vi "LEIN m serial Open Comport.vi"(0 "Comport":refnum<visa-resource-name>, 9 "baud rate (9600)":u32=9600, 11 "error in (no error)":errorcluster, 13 "Reply timeout (1000 ms)":u32=1000) -> (4 "VISA resource name out":refnum<visa-resource-name>, 15 "error out":errorcluster)   [LabVIEW 2011]
doc: "Opner comporten med den valgte VISA ingangen, om error in, gjøre ingenting"
uses:
  <vilib>/Instr/_visa.llb/VISA Configure Serial Port (Instr).vi
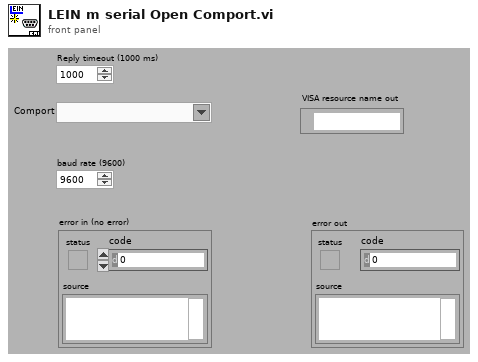
[diagram p1: front panel]
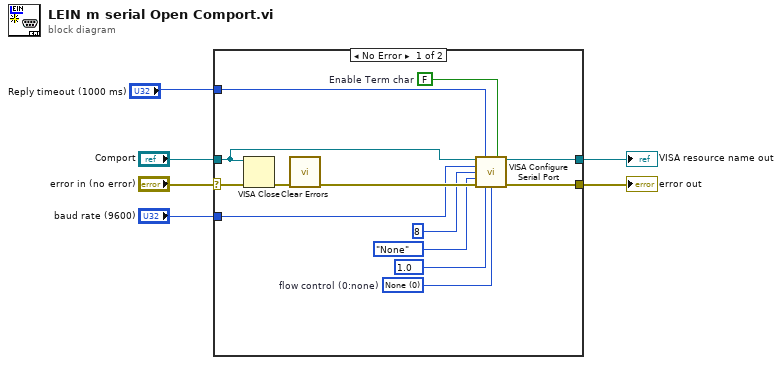
[diagram p0: block diagram]
diagram:
  n1 = case shown="No Error" "error in (no error)" {
    selector: "error in (no error)" -> [w15 w20]
    tunnel: [w18 w21] -> w6
    tunnel: [w17 w20] -> w5
    tunnel: "Comport" -> [w12 w21]
    tunnel: "Reply timeout (1000 ms)" -> [w11 _]
    tunnel: "baud rate (9600)" -> [w10 _]
    frame No Error {
      w9 = u16 10 items=["1.0"=10, "1.5"=15, "2.0"=20] ("stop bits (10: 1 bit)")
      w19 = FALSE  # Enable Term char
      w16 = u16 0 items=["None", "XON/XOFF", "RTS/CTS", "XON/XOFF & RTS/CTS", "DTR/DSR", "XON/XOFF & DTR/DSR"]  # flow control (0:none)
      n2 = VISA Close(VISA resource name=w12, error in (no error)=w15) -> (error out=w14:errorcluster)
      n3 = call <vilib>:"Clear Errors.vi"("error in (no error)"=w14) -> ("error out"=w13:errorcluster)  [unwired: 6 in]
      n4 = call-poly "VISA Configure Serial Port"("VISA resource name"=w12, "timeout (10sec)"=w11, "Enable Termination\nChar (T)"=w19, "baud rate (9600)"=w10, "data bits (8)"=u16 8, "parity (0:none)"=enum16{"None", "Odd", "Even", "Mark", "Space"}."None", "error in (no error)"=w13, "stop bits (10: 1 bit)"=w9, "flow control (0:none)"=w16) -> ("VISA resource name out"=w18:refnum<visa-resource-name>, "error out"=w17:errorcluster)  [unwired: 5 in]
    }
    frame Error {
    }
  }
  "VISA resource name out" <- w6
  "error out" <- w5
